vi "AUTON_Index.vi"(0 "Auton Array":dbl[][](array[numeric]), 5 "MeasuredHeading":dbl, 7 "LeftEncoder":dbl, 9 "RightEncoder":dbl) -> (4 "Right Drive":dbl, 6 "Left Drive":dbl, 8 "Shooter Elevation":dbl, 10 "Shooter Wheel F":dbl, 15 "Shooter Wheel B":dbl)   [LabVIEW 2012]
uses:
  Robot Global Data.vi
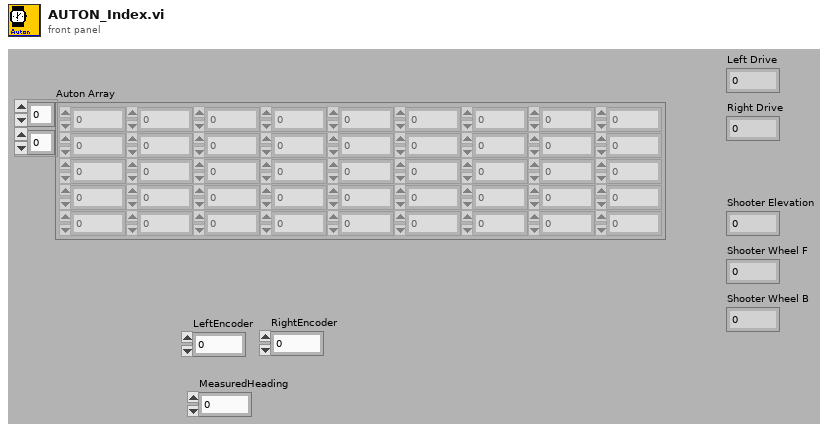
[diagram p1: front panel]
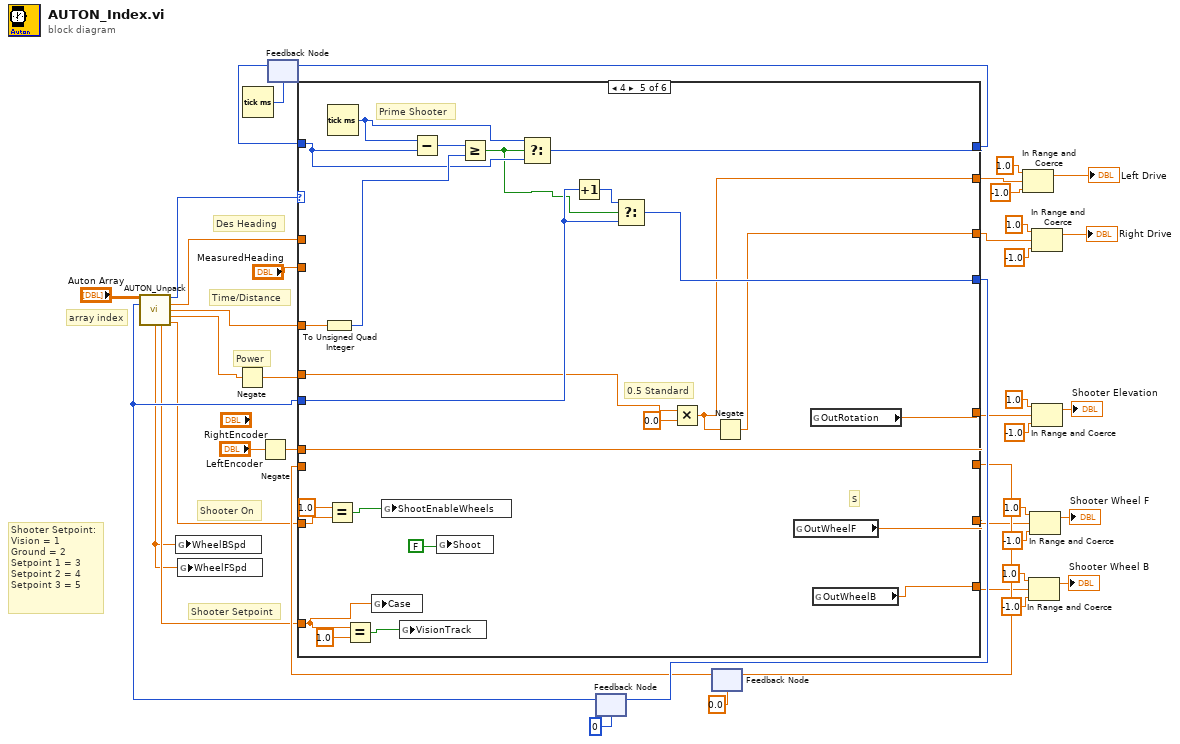
[diagram p0: block diagram]
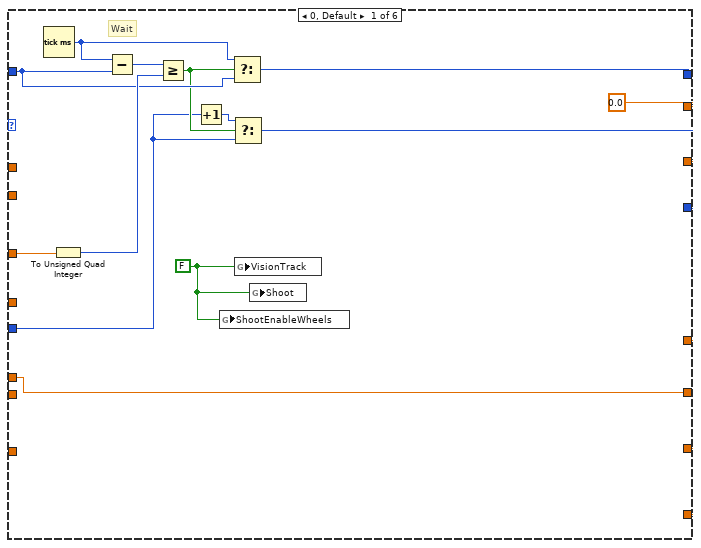
[diagram p2: hidden frame]
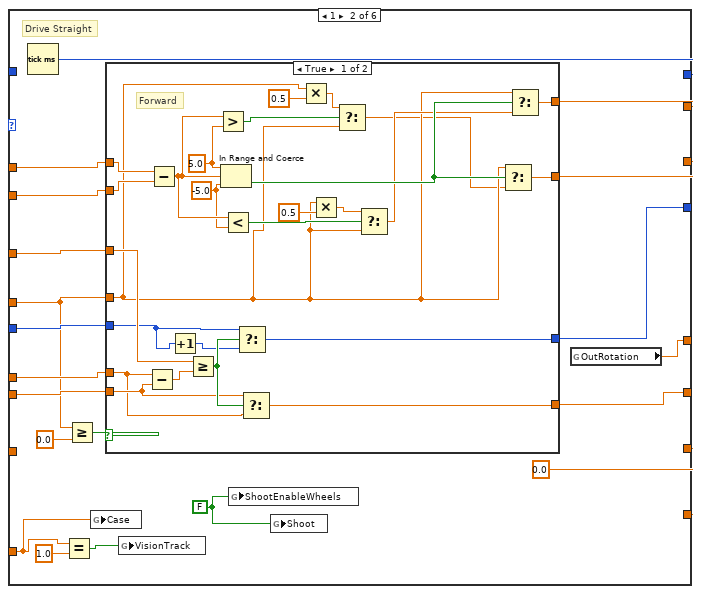
[diagram p3: hidden frame]
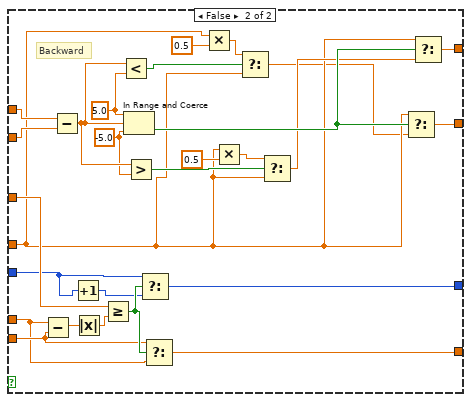
[diagram p4: hidden frame]
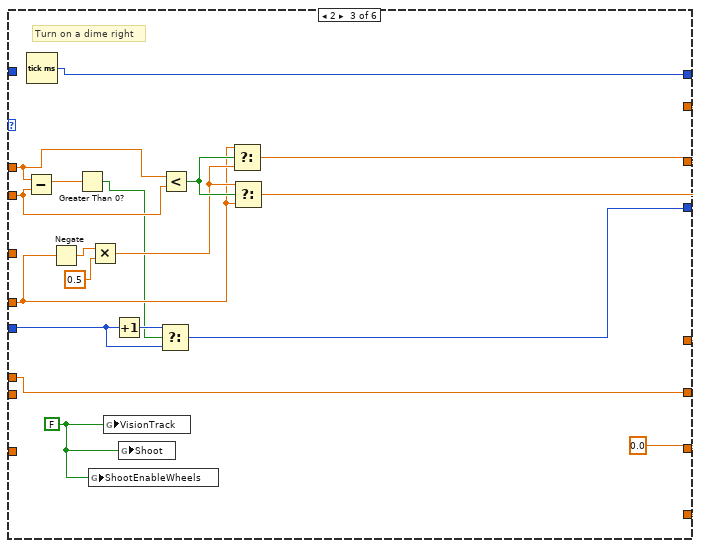
[diagram p5: hidden frame]
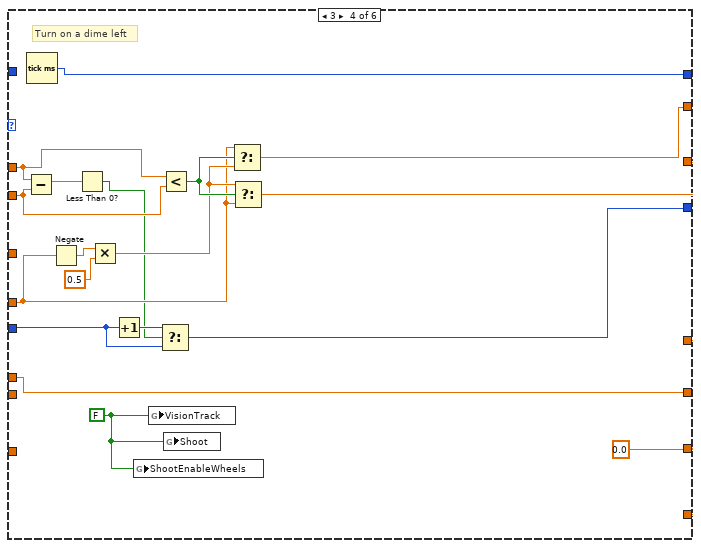
[diagram p6: hidden frame]
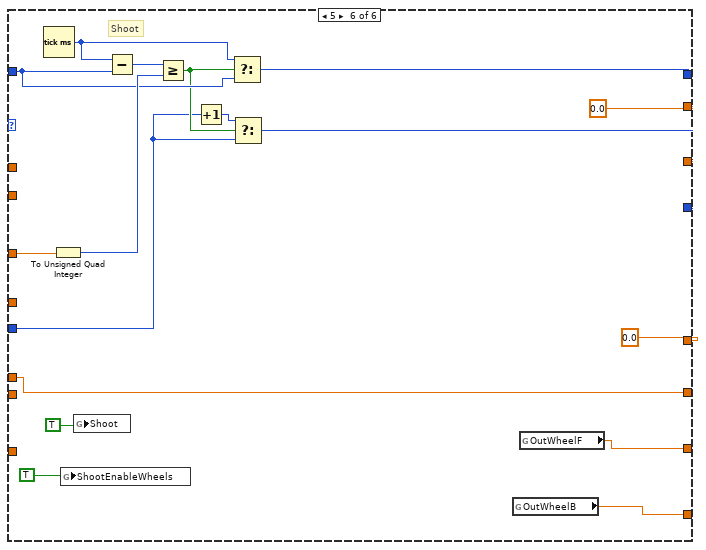
[diagram p7: hidden frame]
diagram:
  # "Shooter Setpoint:\nVision = 1\nGround = 2\nSetpoint 1 = 3\nSetpoint 2 = 4\nSetpoint 3 = 5"
  # "Shooter On"
  # "Shooter Setpoint"
  # "Des Heading"
  # "Time/Distance"
  # "Power"
  # "array index"
  n1 = Tick Count (ms)() -> (millisecond timer value=w39:u32)
  n2 = Negate(x="LeftEncoder") -> (-x=w2:dbl)
  n3 = feedback #1(w39) -> (w40:u32)
  n4 = feedback #2(0) -> (w20:i32)
  n5 = call "AUTON_Unpack.vi"("all rows"="Auton Array", "Index"=w20) -> ("Primitive ID"=w23:i16, "Desired Heading"=w22:dbl, "Time/Distance"=w21:dbl, "Power"=w5:dbl, "Shooter Speed"=w1:dbl, "Shooter Case"=w6:dbl, "Shooter On"=w19:dbl)  [unwired: 6 in, 1 out]
  n6 = global write "Robot Global Data.vi" "WheelBSpd"(w1) -> ()
  n7 = global write "Robot Global Data.vi" "WheelFSpd"(w1) -> ()
  n8 = Negate(x=w5) -> (-x=w4:dbl)
  n9 = feedback #3(0.0) -> (w25:dbl)
  n10 = case shown="4" w23 {
    tunnel: [w46 w72 w140 w158 w187 w197] -> w27
    tunnel: w20 -> [w47 w67 w143 w161 w178 w198]
    tunnel: [w54 w64 w145 w163 w176 w205] -> w29
    tunnel: w40 -> [w51 _ _ _ w177 w202]
    tunnel: w21 -> [w45 w73 _ _ w179 w196]
    tunnel: w22 -> [_ w71 w138 w156 _ _]
    tunnel: [w42 w69 w141 w159 w172 w195] -> w37
    tunnel: [w42 w68 w142 w160 w171 w195] -> w30
    tunnel: w4 -> [_ w63 w132 w150 w173 _]
    tunnel: w2 -> [w43 w65 w139 w157 w188 w193]
    tunnel: "MeasuredHeading" -> [_ w70 w137 w155 _ _]
    tunnel: w25 -> [_ w66 _ _ _ _]
    tunnel: [w43 w74 w139 w157 w188 w193] -> w24
    tunnel: w19 -> [_ _ _ _ w169 _]
    tunnel: w6 -> [_ w57 _ _ w183 _]
    tunnel: [w42 w55 w129 w146 w165 w189] -> w9
    tunnel: [w42 w55 w129 w146 w166 w190] -> w8
    tunnel: [w42 w56 w129 w146 w175 0.0 ("ShootOutElev")] -> w7
    frame 0, Default {
      w44 = FALSE ("ShootTrackEnable")
      w42 = 0.0 ("Numeric")
      # "Wait"
      n11 = Tick Count (ms)() -> (millisecond timer value=w50:u32)
      n12 = To Unsigned Quad Integer(1:w45) -> (0:w52:u64)
      n13 = Subtract(x=w50, y=w51) -> (x-y=w53:u32)
      n14 = Greater Or Equal?(x=w53, y=w52) -> (x >= y?=w49:bool)
      n15 = Increment(x=w47) -> (x+1=w48:i32)
      n16 = global write "Robot Global Data.vi" "ShootEnableWheels"(w44) -> ()
      n17 = Select(t=w50, s=w49, f=w51) -> (s? t:f=w54:u32)
      n18 = Select(t=w48, s=w49, f=w47) -> (s? t:f=w46:i32)
      n19 = global write "Robot Global Data.vi" "VisionTrack"(w44) -> ()
      n20 = global write "Robot Global Data.vi" "Shoot"(w44) -> ()
    }
    frame 1 {
      w60 = FALSE ("ShootTrackEnable")
      w55 = 0.0 ("Numeric")
      # "Drive Straight"
      n21 = Tick Count (ms)() -> (millisecond timer value=w64:u32)
      n22 = Equal?(x=w57, y=1.0) -> (x = y?=w58:bool)
      n23 = Greater Or Equal?(x=w63, y=0.0) -> (x >= y?=w61:bool)
      n24 = global write "Robot Global Data.vi" "Case"(w57) -> ()
      n25 = case shown="True" w61 {
        tunnel: [w100 w127] -> w74
        tunnel: w73 -> [w98 w126]
        tunnel: [w96 w124] -> w72
        tunnel: w71 -> [w95 w123]
        tunnel: w70 -> [w94 w122]
        tunnel: [w92 w120] -> w69
        tunnel: [w91 w119] -> w68
        tunnel: w63 -> [w80 w108]
        tunnel: w67 -> [w77 w105]
        tunnel: w66 -> [w76 w104]
        tunnel: w65 -> [w75 w103]
        frame True {
          w88 = -5.0 ("lower limit")
          w90 = 5.0 ("upper limit")
          # "Forward"
          n26 = Subtract(x=w75, y=w76) -> (x-y=w99:dbl)
          n27 = Subtract(x=w95, y=w94) -> (x-y=w89:dbl)
          n28 = Increment(x=w77) -> (x+1=w78:i32)
          n29 = Greater Or Equal?(x=w98, y=w99) -> (x >= y?=w97:bool)
          n30 = Greater?(x=w89, y=w90) -> (0:w83:bool)
          n31 = In Range and Coerce(upper limit=w90, x=w89, lower limit=w88) -> (In Range?=w93:bool)  [unwired: 1 out]
          n32 = Less?(x=w89, y=w88) -> (x < y?=w87:bool)
          n33 = Select(t=w77, s=w97, f=w78) -> (s? t:f=w96:i32)
          n34 = Select(t=w76, s=w97, f=w75) -> (s? t:f=w100:dbl)
          n35 = Multiply(x=w80, y=0.5) -> (x*y=w82:dbl)
          n36 = Multiply(x=w80, y=0.5) -> (x*y=w85:dbl)
          n37 = Select(t=w82, s=w83, f=w80) -> (s? t:f=w79:dbl)
          n38 = Select(t=w85, s=w87, f=w80) -> (s? t:f=w84:dbl)
          n39 = Select(t=w80, s=w93, f=w79) -> (s? t:f=w91:dbl)
          n40 = Select(t=w80, s=w93, f=w84) -> (s? t:f=w92:dbl)
        }
        frame False {
          w116 = -5.0 ("lower limit")
          w118 = 5.0 ("upper limit")
          # "Backward"
          n41 = Subtract(x=w103, y=w104) -> (x-y=w101:dbl)
          n42 = Subtract(x=w123, y=w122) -> (x-y=w117:dbl)
          n43 = Increment(x=w105) -> (x+1=w106:i32)
          n44 = Absolute Value(x=w101) -> (abs(x)=w102:dbl)
          n45 = Greater Or Equal?(x=w126, y=w102) -> (x >= y?=w125:bool)
          n46 = Less?(x=w117, y=w118) -> (x < y?=w111:bool)
          n47 = In Range and Coerce(upper limit=w118, x=w117, lower limit=w116) -> (In Range?=w121:bool)  [unwired: 1 out]
          n48 = Greater?(x=w117, y=w116) -> (0:w115:bool)
          n49 = Select(t=w105, s=w125, f=w106) -> (s? t:f=w124:i32)
          n50 = Select(t=w104, s=w125, f=w103) -> (s? t:f=w127:dbl)
          n51 = Multiply(x=w108, y=0.5) -> (x*y=w110:dbl)
          n52 = Multiply(x=w108, y=0.5) -> (x*y=w113:dbl)
          n53 = Select(t=w110, s=w111, f=w108) -> (s? t:f=w107:dbl)
          n54 = Select(t=w113, s=w115, f=w108) -> (s? t:f=w112:dbl)
          n55 = Select(t=w108, s=w121, f=w107) -> (s? t:f=w119:dbl)
          n56 = Select(t=w108, s=w121, f=w112) -> (s? t:f=w120:dbl)
        }
      }
      n57 = global write "Robot Global Data.vi" "VisionTrack"(w58) -> ()
      n58 = global write "Robot Global Data.vi" "ShootEnableWheels"(w60) -> ()
      n59 = global write "Robot Global Data.vi" "Shoot"(w60) -> ()
      n60 = global read "Robot Global Data.vi" "OutRotation"() -> (w56:dbl)
    }
    frame 2 {
      w128 = FALSE ("ShootTrackEnable")
      w129 = 0.0 ("Numeric")
      # "Turn on a dime right"
      n61 = Subtract(x=w138, y=w137) -> (x-y=w131:dbl)
      n62 = Tick Count (ms)() -> (millisecond timer value=w145:u32)
      n63 = Negate(x=w132) -> (-x=w135:dbl)
      n64 = Greater Than 0?(x=w131) -> (x > 0?=w130:bool)
      n65 = global write "Robot Global Data.vi" "ShootEnableWheels"(w128) -> ()
      n66 = Multiply(x=w135, y=0.5) -> (x*y=w133:dbl)
      n67 = global write "Robot Global Data.vi" "VisionTrack"(w128) -> ()
      n68 = Increment(x=w143) -> (x+1=w144:i32)
      n69 = global write "Robot Global Data.vi" "Shoot"(w128) -> ()
      n70 = Select(t=w144, s=w130, f=w143) -> (s? t:f=w140:i32)
      n71 = Less?(x=w138, y=w137) -> (x < y?=w136:bool)
      n72 = Select(t=w132, s=w136, f=w133) -> (s? t:f=w141:dbl)
      n73 = Select(t=w133, s=w136, f=w132) -> (s? t:f=w142:dbl)
    }
    frame 3 {
      w147 = FALSE ("ShootTrackEnable")
      w146 = 0.0 ("Numeric")
      # "Turn on a dime left"
      n74 = Subtract(x=w156, y=w155) -> (x-y=w149:dbl)
      n75 = Tick Count (ms)() -> (millisecond timer value=w163:u32)
      n76 = Negate(x=w150) -> (-x=w153:dbl)
      n77 = Less Than 0?(x=w149) -> (x < 0?=w148:bool)
      n78 = Multiply(x=w153, y=0.5) -> (x*y=w151:dbl)
      n79 = Increment(x=w161) -> (x+1=w162:i32)
      n80 = global write "Robot Global Data.vi" "ShootEnableWheels"(w147) -> ()
      n81 = global write "Robot Global Data.vi" "VisionTrack"(w147) -> ()
      n82 = Select(t=w162, s=w148, f=w161) -> (s? t:f=w158:i32)
      n83 = Less?(x=w156, y=w155) -> (x < y?=w154:bool)
      n84 = global write "Robot Global Data.vi" "Shoot"(w147) -> ()
      n85 = Select(t=w150, s=w154, f=w151) -> (s? t:f=w159:dbl)
      n86 = Select(t=w151, s=w154, f=w150) -> (s? t:f=w160:dbl)
    }
    frame 4 {
      # "S"
      # "0.5 Standard"
      # "Prime Shooter"
      n87 = To Unsigned Quad Integer(1:w179) -> (0:w181:u64)
      n88 = Equal?(x=1.0, y=w169) -> (x = y?=w167:bool)
      n89 = Tick Count (ms)() -> (millisecond timer value=w180:u32)
      n90 = Equal?(x=w183, y=1.0) -> (x = y?=w184:bool)
      n91 = global write "Robot Global Data.vi" "Case"(w183) -> ()
      n92 = global write "Robot Global Data.vi" "ShootEnableWheels"(w167) -> ()
      n93 = global write "Robot Global Data.vi" "VisionTrack"(w184) -> ()
      n94 = Subtract(x=w180, y=w177) -> (x-y=w182:u32)
      n95 = global write "Robot Global Data.vi" "Shoot"(FALSE ("Shoot")) -> ()
      n96 = Greater Or Equal?(x=w182, y=w181) -> (x >= y?=w174:bool)
      n97 = Select(t=w180, s=w174, f=w177) -> (s? t:f=w176:u32)
      n98 = Increment(x=w178) -> (x+1=w186:i32)
      n99 = Select(t=w186, s=w174, f=w178) -> (s? t:f=w187:i32)
      n100 = Multiply(x=w173, y=0.0) -> (x*y=w172:dbl)
      n101 = Negate(x=w172) -> (-x=w171:dbl)
      n102 = global read "Robot Global Data.vi" "OutWheelF"() -> (w166:dbl)
      n103 = global read "Robot Global Data.vi" "OutRotation"() -> (w175:dbl)
      n104 = global read "Robot Global Data.vi" "OutWheelB"() -> (w165:dbl)
    }
    frame 5 {
      w195 = 0.0 ("Numeric")
      # "Shoot"
      n105 = Tick Count (ms)() -> (millisecond timer value=w201:u32)
      n106 = To Unsigned Quad Integer(1:w196) -> (0:w203:u64)
      n107 = global write "Robot Global Data.vi" "ShootEnableWheels"(TRUE ("ShootEnableWheels")) -> ()
      n108 = global write "Robot Global Data.vi" "Shoot"(TRUE ("Shoot")) -> ()
      n109 = Subtract(x=w201, y=w202) -> (x-y=w204:u32)
      n110 = Greater Or Equal?(x=w204, y=w203) -> (x >= y?=w200:bool)
      n111 = Increment(x=w198) -> (x+1=w199:i32)
      n112 = Select(t=w201, s=w200, f=w202) -> (s? t:f=w205:u32)
      n113 = Select(t=w199, s=w200, f=w198) -> (s? t:f=w197:i32)
      n114 = global read "Robot Global Data.vi" "OutWheelB"() -> (w189:dbl)
      n115 = global read "Robot Global Data.vi" "OutWheelF"() -> (w190:dbl)
    }
  }
  n116 = feedback-in #1(w29) -> ()
  n117 = feedback-in #2(w27) -> ()
  n118 = feedback-in #3(w24) -> ()
  n119 = In Range and Coerce(upper limit=1.0, x=w37, lower limit=-1.0) -> (coerced(x)=→"Left Drive":dbl)  [unwired: 1 out]
  n120 = In Range and Coerce(upper limit=1.0, x=w9, lower limit=-1.0) -> (coerced(x)=→"Shooter Wheel B":dbl)  [unwired: 1 out]
  n121 = In Range and Coerce(upper limit=1.0, x=w8, lower limit=-1.0) -> (coerced(x)=→"Shooter Wheel F":dbl)  [unwired: 1 out]
  n122 = In Range and Coerce(upper limit=1.0, x=w30, lower limit=-1.0) -> (coerced(x)=→"Right Drive":dbl)  [unwired: 1 out]
  n123 = In Range and Coerce(upper limit=1.0, x=w7, lower limit=-1.0) -> (coerced(x)=→"Shooter Elevation":dbl)  [unwired: 1 out]
